vi "tb_transfer to 2x clock (U512 to U256).vi"() -> ()   [LabVIEW 2012]
uses:
  <vilib>/Platform/TimedLoop/XDataNode/timing_clust.ctl
  <vilib>/Platform/TimedLoop/XDataNode/nitl_modes.ctl
  <vilib>/Platform/TimedLoop/XDataNode/wakeup.ctl
  <vilib>/rvi/Emulation/niFpgaSctlEmulationRegisterWithScheduler.vi
  <vilib>/rvi/Emulation/niFpgaSctlEmulationScheduler.vi
  <vilib>/rvi/FIFO/Fifo_Resource/nirvififoEmulationSetSize.vi
  <vilib>/rvi/DataTransferAndStorage/Container/Common/niFpgaContainerGetUniqueNameForEmu.vi
  <vilib>/rvi/errors/niFpgaSetErrorForExecOnDevCompSimple.vi
  <vilib>/rvi/eio/common/nirviEmuReportErrorAndStop.vi
  <vilib>/rvi/Emulation/niFpgaSctlEmulationFifoFullMgr.vi
  <vilib>/rvi/Emulation/niFpgaSctlEmulationResourceMgr.vi
  <vilib>/Platform/TimedLoop/XDataNode/XDataNode.xnode
  <vilib>/rvi/DataTransferAndStorage/Container/XNode/niFpgaContainer.xnode
  <vilib>/rvi/FIFO/Fifo_Resource/nirvififoEmulationGetNumberOfElementsToWrite.vi
  <vilib>/rvi/FIFO/Fifo_Resource/nirvififoEmulationWrite.vi
  <vilib>/Platform/TimedLoop/XDataNode/XDNodeRunTimeDep.lvlib
panel:
  out "Data":i16(graph)
  out "Collected Data":u64[](array[numeric])
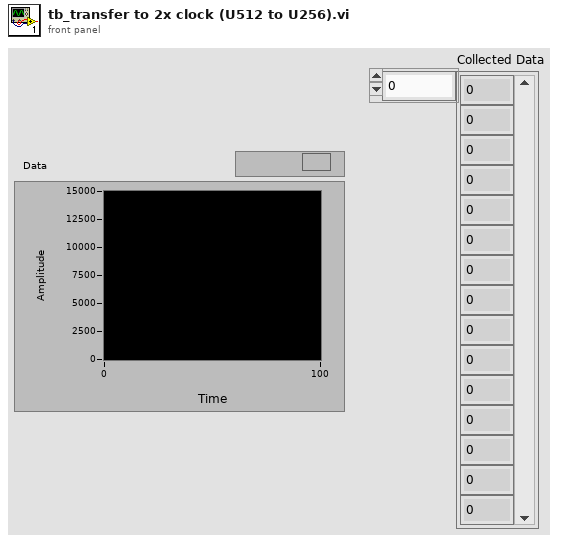
[diagram p1: front panel]
types:
  T1 = typedef "XDNodeRunTimeDep.lvlib/timing_clust.ctl" = cluster{"Expected End [f-1]":u64, "Actual End [f-1]":u64, "Finished Late? [f-1]":bool, "Expected End [i-1]":u64, "Actual End [i-1]":u64, "Finished Late? [i-1]":bool, "Expected Start [i]":u64, "Actual Start [i]":u64, "Expected Start [f]":u64, "Actual Start [f]":u64, "Source Name":string, "Structure Name":string, "Period":i64, "Deadline":i64, "Offset":i64, "Start":i64, "Priority":i32, "Timeout":i32, "Mode":T2, "Wakeup Reason":T3, "Error":errorcluster, "Source Type":string, "Secondary Source Type":string, "Global End Time":u64, "Global Start Time":u64, "Frame Duration":u64, "Iteration Duration":u64, "Assigned CPU":i32, "I/O Scan Engine Mode":u32}
  T2 = typedef "XDNodeRunTimeDep.lvlib/nitl_modes.ctl" = enum32{"No Change", "Process missed periods, maintain original phase", "Discard missed periods, maintain original phase", "Process missed periods, ignore original phase", "Discard missed periods, ignore original phase"}
  T3 = typedef "XDNodeRunTimeDep.lvlib/wakeup.ctl" = enum32{"Normal", "Aborted", "Asynchronous wakeup", "Timing source error", "Timed loop error", "Timeout"}
  T4 = cluster{"U64.0":u64, "U64.1":u64, "U64.2":u64, "U64.3":u64}
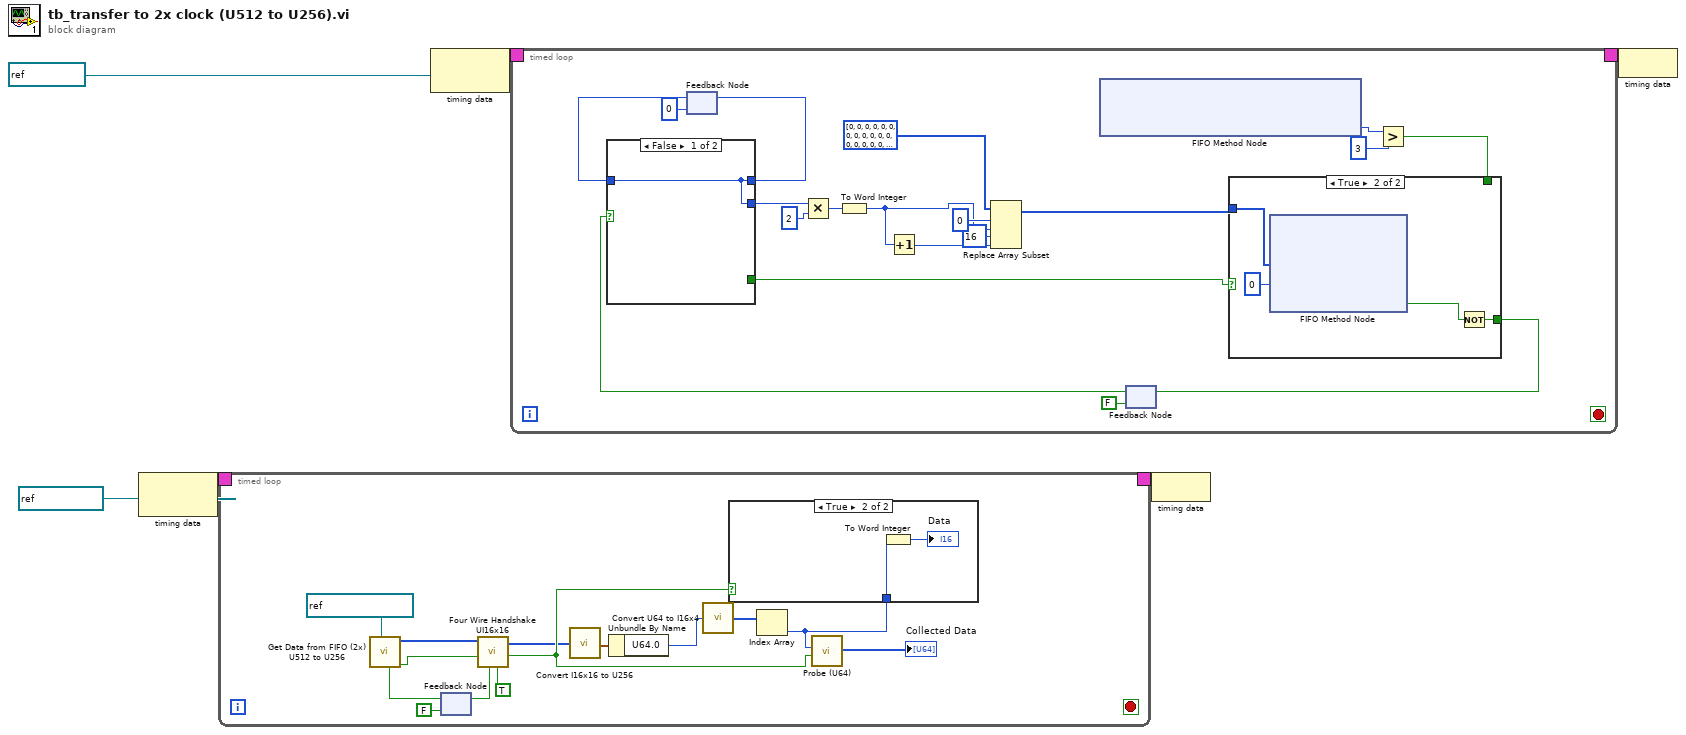
[diagram p0: block diagram]
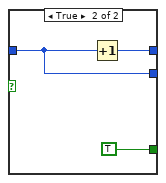
[diagram p3: hidden frame]
diagram:
  n1 = node-c288(refnum<k21> "100MHz" ("Source Name")) -> (w4:T1)
  n2 = timed-loop {
    timing: w4 -> [_]
    timing-out: [_] -> w3
    stop <- _ stop-if-true
    n3 = feedback #1(FALSE ("ready for input")) -> (w17:bool)
    n4 = call <userlib>:"Get Data from FIFO (2x) U512 to U256.vi"("Ready for Output"=w17, "FIFO In"=refnum<k21> "FIFO (U512)") -> ("Data Valid"=w16:bool, "Output Data"=w14:i16[])  [unwired: 8 in]
    n5 = call <instrlib>:"Four Wire Handshake UI16x16.vi"("ready for output"=TRUE, "data valid"=w16, "Data"=w14) -> ("valid out"=w12:bool, "Data Out"=w7:i16[], "ready for input"=w18:bool)  [unwired: 5 in, 1 out]
    n6 = feedback-in #1(w18) -> ()
    n7 = call <userlib>:"Convert I16x16 to U256.vi"("I16x16 Data"=w7) -> ("U64x4 CLuster"=w13:T4)  [unwired: 14 in]
    n8 = Unbundle By Name(w13) -> ("U64.0"=w10:u64)
    n9 = call <userlib>:"Convert U64 to I16x4.vi"("U64"=w10) -> ("4xI16 Array"=w11:u16[])  [unwired: 14 in]
    n10 = Index Array(array=w11) -> (element=w9:u16)  [unwired: 1 in]
    n11 = case shown="True" w12 {
      tunnel: w9 -> [_ w22]
      frame False {
      }
      frame True {
        n12 = To Word Integer(number=w22) -> (16bit integer=→"Data":i16)
      }
    }
    n13 = call <userlib>:"Probe (U64).vi"("Data Valid"=w12, "Input Data"=w9) -> ("Collected Data"=→"Collected Data":u64[])  [unwired: 9 in]
  }
  n14 = node-c288(refnum<k21> "50MHz" ("Source Name")) -> (w6:T1)
  n15 = timed-loop {
    timing: w6 -> [_]
    timing-out: [_] -> w5
    stop <- _ stop-if-true
    n16 = feedback #2(u32 0) -> (w42:u32)
    n17 = xnode ("FIFO Method Node")() -> ("Number of Elements to Write"=w34:u32)  [unwired: 1 in, 1 out]
    n18 = feedback #3(FALSE) -> (w36:bool)
    n19 = case shown="False" w36 {
      tunnel: w42 -> [w44 w45]
      tunnel: [w44 w47] -> w40
      tunnel: [_ TRUE] -> w38
      tunnel: [w44 w45] -> w39
      frame False {
      }
      frame True {
        n20 = Increment(x=w45) -> (x+1=w47:u32)
      }
    }
    n21 = feedback-in #2(w40) -> ()
    n22 = Multiply(x=w39, y=u32 2) -> (x*y=w31:u32)
    n23 = To Word Integer(number=w31) -> (16bit integer=w27:i16)
    n24 = Increment(x=w27) -> (x+1=w25:i16)
    n25 = Replace Array Subset(array=i16[] [0, 0, 0, 0, 0, 0, 0, 0, 0, 0, 0, 0, 0, 0, 0, 0, 0, 0, 0, 0, 0, 0, 0, 0, 0, 0, 0, 0, 0, 0, 0, 0], new element #1=w27, index #1=0 ("index"), new element #2=w25, index #2=16 ("index")) -> (w29:i16[])
    n26 = Greater?(x=w34, y=u32 3) -> (0:w32:bool)
    n27 = case shown="True" w38 {
      tunnel: w29 -> [_ w49]
      tunnel: [w48 w51] -> w37
      tunnel: w32 -> [w48 _]
      frame False {
      }
      frame True {
        n28 = xnode ("FIFO Method Node")("Element"=w49, "Timeout"=0) -> ("Timed Out?"=w52:bool)  [unwired: 1 in, 1 out]
        n29 = Not(x=w52) -> (.not. x?=w51:bool)
      }
    }
    n30 = feedback-in #3(w37) -> ()
  }
  n31 = node-c288(w3) -> ()
  n32 = node-c288(w5) -> ()
